vi "MasterFrame.vi"(8 "数组大小":i32, 9 "Mode":bool, 10 "buf":u8[](array[numeric]) format="%02x") -> (1 "接收显示":string, 2 "数据帧分析":string)   [LabVIEW 2015]
doc: "Mode = 1? RTU；ASCII;"
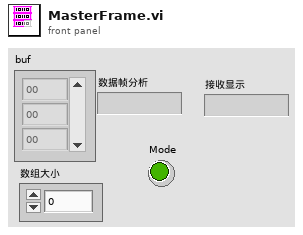
[diagram p1: front panel]
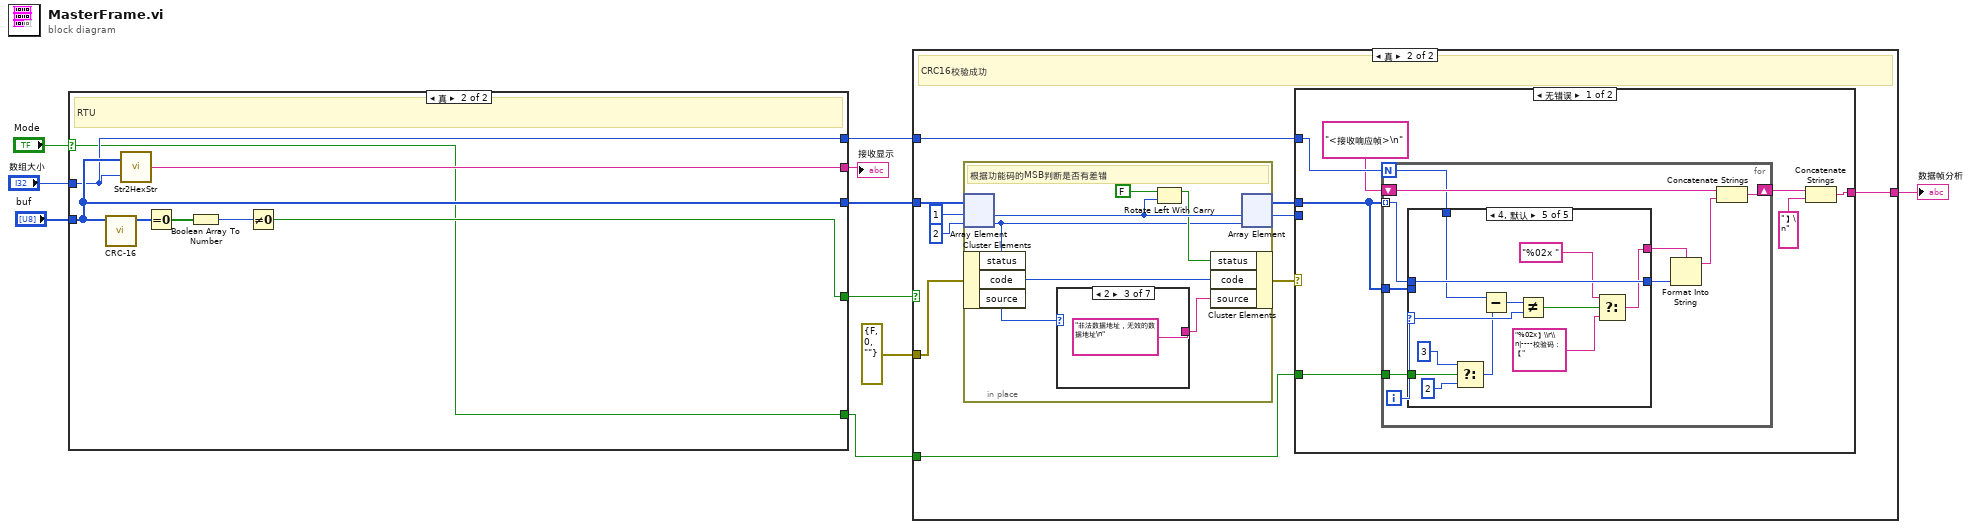
[diagram p0: block diagram]
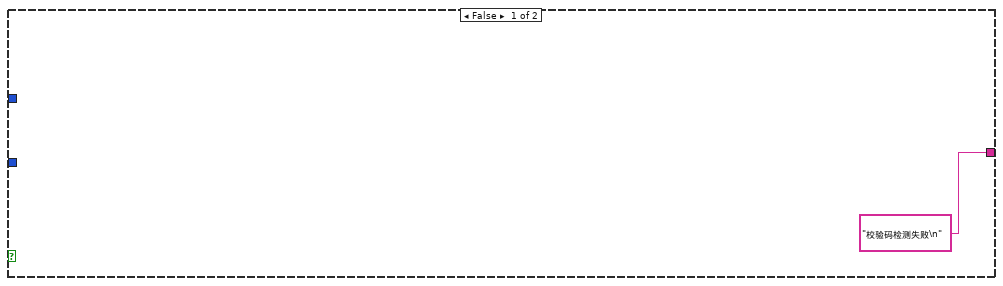
[diagram p2: hidden frame]
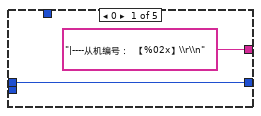
[diagram p3: hidden frame]
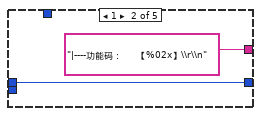
[diagram p4: hidden frame]
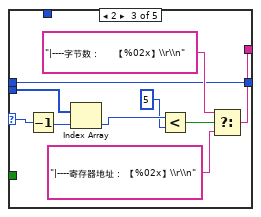
[diagram p5: hidden frame]
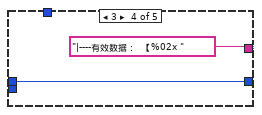
[diagram p6: hidden frame]
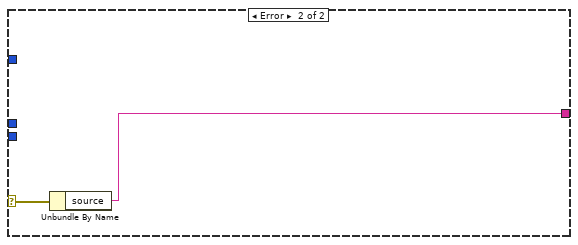
[diagram p7: hidden frame]
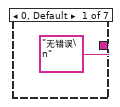
[diagram p8: hidden frame]
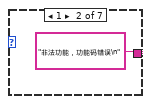
[diagram p9: hidden frame]
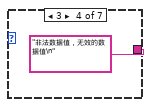
[diagram p10: hidden frame]
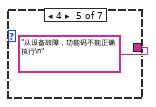
[diagram p11: hidden frame]
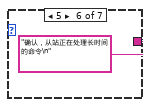
[diagram p12: hidden frame]
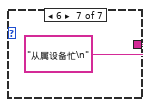
[diagram p13: hidden frame]
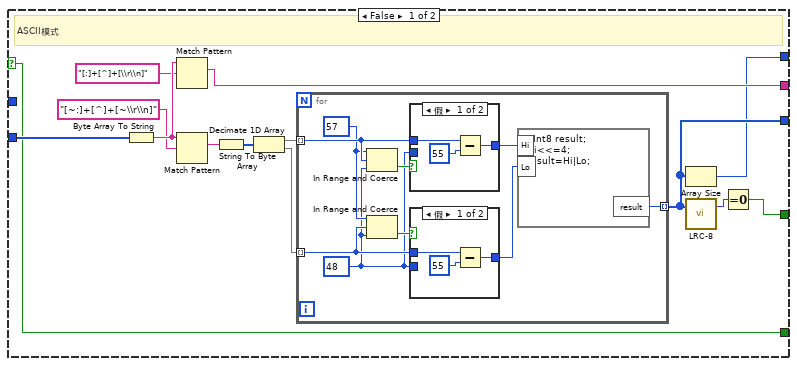
[diagram p14: hidden frame]
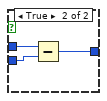
[diagram p15: hidden frame]
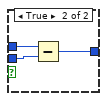
[diagram p16: hidden frame]
diagram:
  n1 = case shown="真" "Mode" {
    selector: "Mode" -> [w11 w46]
    tunnel: "buf" -> [w24 w48]
    tunnel: "数组大小" -> [_ w47]
    tunnel: [w15 w50] -> w9
    tunnel: [w14 w49] -> w8
    tunnel: [w13 w48] -> w7
    tunnel: [w12 w47] -> w4
    tunnel: [w11 w46] -> w1
    frame False {
      # "ASCII模式"
      n2 = Byte Array To String(unsigned byte array=w24) -> (string=w23:string)
      n3 = Match Pattern(string=w23, regular expression="[:]+[^]+[\\r\\n]") -> (match substring=w15:string)  [unwired: 1 in, 3 out]
      n4 = Match Pattern(string=w23, regular expression="[~:]+[^]+[~\\r\\n]") -> (match substring=w18:string)  [unwired: 1 in, 3 out]
      n5 = String To Byte Array(string=w18) -> (unsigned byte array=w21:u8[])
      n6 = Decimate 1D Array(w21) -> (w20:u8[], w19:u8[])
      n7 = for {
        tunnel: w20 -> [w32] mode=indexing
        tunnel: w19 -> [w30] mode=indexing
        tunnel: [w25] -> w13 mode=indexing
        w29 = u8 57
        w28 = u8 48
        n8 = In Range and Coerce(upper limit=w29, x=w32, lower limit=w28) -> (In Range?=w33:bool)  [unwired: 1 out]
        n9 = In Range and Coerce(upper limit=w29, x=w30, lower limit=w28) -> (In Range?=w31:bool)  [unwired: 1 out]
        n10 = case shown="假" w33 {
          tunnel: w32 -> [w41 w45]
          tunnel: w28 -> [_ w44]
          tunnel: [w40 w43] -> w27
          frame False {
            n11 = Subtract(x=w41, y=u8 55) -> (x-y=w40:u8)
          }
          frame True {
            n12 = Subtract(x=w45, y=w44) -> (x-y=w43:u8)
          }
        }
        n13 = case shown="假" w31 {
          tunnel: w30 -> [w35 w39]
          tunnel: [w34 w38] -> w26
          tunnel: w28 -> [_ w37]
          frame False {
            n14 = Subtract(x=w35, y=u8 55) -> (x-y=w34:u8)
          }
          frame True {
            n15 = Subtract(x=w39, y=w37) -> (x-y=w38:u8)
          }
        }
        n16 = formula code="uInt8 result;\nHi<<=4;\nresult=Hi|Lo;"("Hi"=w27, "Lo"=w26) -> ("result"=w25:u8)
      }
      n17 = Array Size(array=w13) -> (size(s)=w12:i32)
      n18 = call "LRC-8.vi"("Frame in"=w13) -> ("LRC-8"=w16:u8)  [unwired: 2 in]
      n19 = Equal To 0?(x=w16) -> (x = 0?=w14:bool)
    }
    frame True {
      # "RTU"
      n20 = call "CRC-16.vi"("Frame in"=w48) -> ("CRC-16"=w53:u8[])  [unwired: 6 in]
      n21 = call "Str2HexStr.vi"("数组大小"=w47, "数组"=w48) -> ("OutStr"=w50:string)
      n22 = Equal To 0?(x=w53) -> (x = 0?=w52:bool[])
      n23 = Boolean Array To Number(Boolean array=w52) -> (number=w51:u32)
      n24 = Not Equal To 0?(x=w51) -> (x != 0?=w49:bool)
    }
  }
  "接收显示" <- w9
  n25 = case shown="真" w8 {
    tunnel: w7 -> [_ w64]
    tunnel: errorcluster {"status"=FALSE, "code"=0, "source"=""} ("错误常量") -> [_ w62]
    tunnel: ["校验码检测失败\n" w58] -> w3
    tunnel: w4 -> [_ w56]
    tunnel: w1 -> [_ w55]
    frame False {
    }
    frame True {
      # "CRC16校验成功"
      n26 = in-place {
        # "根据功能码的MSB判断是否有差错"
        n27 = in-place-array #1(w64, 1, 2) -> (w116:u8, w113:u8)
        n28 = in-place-cluster #2(w62) -> ()  [unwired: 3 out]
        n29 = case shown="2" w113 {
          tunnel: ["无错误\n" "非法功能，功能码错误\n" "非法数据地址，无效的数据地址\n" "非法数据值，无效的数据值\n" "从设备故障，功能码不能正确执行\n" "确认，从站正在处理长时间的命令\n" "从属设备忙\n"] -> w112
          frame 0, Default {
          }
          frame 1 {
          }
          frame 2 {
          }
          frame 3 {
          }
          frame 4 {
          }
          frame 5 {
          }
          frame 6 {
          }
        }
        n30 = Rotate Left With Carry(2:w116, 3:FALSE) -> (1:w114:bool)  [unwired: 1 out]
        n31 = in-place-cluster #2("status"=w114, "code"=w113, "source"=w112) -> (w60:errorcluster)
        n32 = in-place-array #1(w116, w113) -> (w57:u8[], w59:i32)  [unwired: 1 out]
      }
      n33 = case shown="无错误" w60 {
        selector: w60 -> [_ w111]
        tunnel: [w70 w110] -> w58
        tunnel: w57 -> [w71 _]
        tunnel: w59 -> [_ _]
        tunnel: w56 -> [w69 _]
        tunnel: w55 -> [w65 _]
        frame No Error {
          n34 = for {
            N: w69 -> [w73]
            shift-right: [w81] -> w67
            shift-left: "<接收响应帧>\n" -> [w80]
            tunnel: w71 -> [w74] mode=indexing
            tunnel: w71 -> [w76]
            tunnel: w65 -> [w72]
            i -> [w77]
            n35 = case shown="4, 默认" w77 {
              selector: w77 -> [_ _ w95 _ w102]
              tunnel: ["|----从机编号：  【%02x】\\r\\n" "|----功能码：     【%02x】\\r\\n" w88 "|----有效数据：  【%02x " w104] -> w79
              tunnel: w76 -> [_ _ w93 _ _]
              tunnel: [w82 w84 w87 w96 w109] -> w75
              tunnel: w74 -> [w82 w84 w87 w96 w109]
              tunnel: w73 -> [_ _ _ _ w108]
              tunnel: w72 -> [_ _ _ _ w101]
              frame 0 {
              }
              frame 1 {
              }
              frame 2 {
                n36 = Decrement(x=w95) -> (x-1=w94:i32)
                n37 = Index Array(array=w93, index=w94) -> (element=w92:u8)
                n38 = Less?(x=w92, y=u8 5) -> (x < y?=w90:bool)
                n39 = Select(t="|----字节数：     【%02x】\\r\\n", s=w90, f="|----寄存器地址： 【%02x】\\r\\n") -> (s? t:f=w88:string)
              }
              frame 3 {
              }
              frame 4, Default {
                n40 = Select(t=3, s=w101, f=2) -> (s? t:f=w99:i32)
                n41 = Subtract(x=w108, y=w99) -> (x-y=w107:i32)
                n42 = Not Equal?(x=w107, y=w102) -> (x != y?=w106:bool)
                n43 = Select(t="%02x ", s=w106, f="%02x】\\r\\n|----校验码：     【") -> (s? t:f=w104:string)
              }
            }
            n44 = Format Into String(format string=w79, w75) -> (resulting string=w78:string)  [unwired: 2 in, 1 out]
            n45 = Concatenate Strings(w80, w78) -> (w81:string)
          }
          n46 = Concatenate Strings(w67, "】\n") -> (w70:string)
        }
        frame Error {
          n47 = Unbundle By Name(w111) -> ("source"=w110:string)
        }
      }
    }
  }
  "数据帧分析" <- w3
